vi "InitializeMission.vi"(0 "GenericMission in":refnum<class "GenericMission.lvclass">, 1 "Duration (s)":dbl=-1.0, 5 "Mission Type":T2, 7 "ID#":u16, 9 "Points of Interest":T1[](array[typedef]) {"North" format="%#_10f"; "East" format="%#_8f"}, 11 "Error In":errorcluster, 12 "Timeout (s)":dbl=-1.0, 14 "Tolerance (m)":dbl) -> (4 "GenericMission out":refnum<class "GenericMission.lvclass">, 15 "Error Out":errorcluster)   [LabVIEW 2013, in "GenericMission.lvclass"]
doc: "This VI initializes a mission. Mission Type, Points of Interest, and Tolerance are required, and timeout and duration are both optional. This should not need to be overriden by child classes."
uses:
  GenericMission.lvclass
  Data/TypeDefs/MissionTypeControl.ctl
  Data/TypeDefs/UTM Location.ctl
  GenericMission.lvclass/GenericMission.ctl
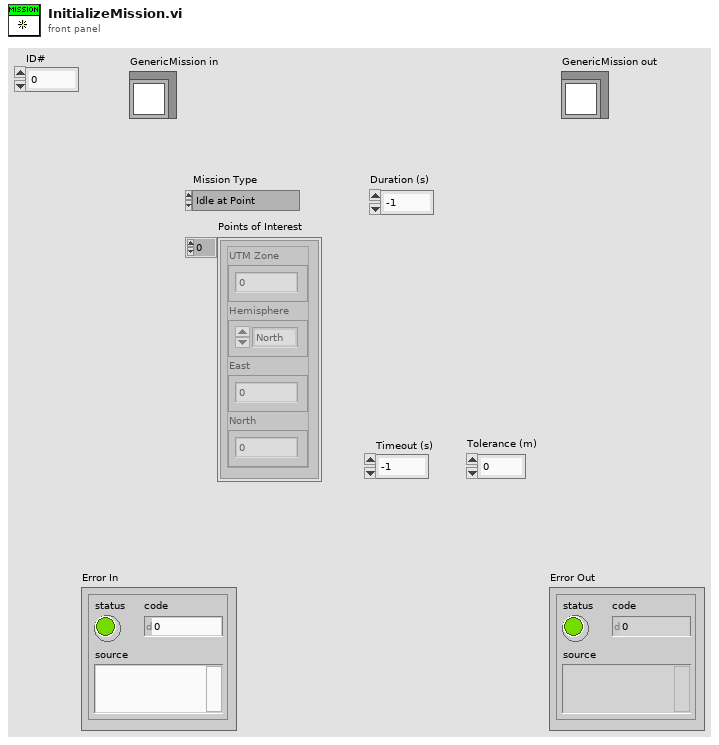
[diagram p1: front panel]
types:
  T1 = typedef "UTM Location.ctl" = cluster{"UTM Zone":dbl, "Hemisphere":enum16{"North", "South"}, "East":dbl, "North":dbl}
  T2 = typedef "MissionTypeControl.ctl" = enum16{"Idle at Point", "Drive to Waypoint", "Round Buoy to Port", "Round Buoy to Starboard", "Pass Between Buoys", "Station Keeping"}
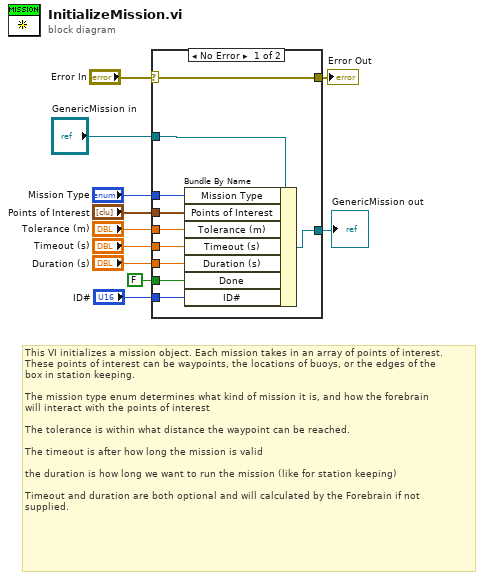
[diagram p0: block diagram]
diagram:
  # "This VI initializes a mission object. Each mission takes in an array of points of interest.\nThese points of interest can be waypoints, the locations of buoys, or the edges of the \nbox in station keeping. \n\nThe mission type enum determines what kind of mission it is, and how the forebrain \nwill interact with the points of interest\n\nThe tolerance is within what distance the waypoint can be reached. \n\nThe timeout is after how long the mission is valid\n\nthe duration is how long we want to run the mission (like for station keeping)\n\nTimeout and duration are both optional and will calculated by the Forebrain if not \nsupplied."
  n1 = case shown="No Error" "Error In" {
    selector: "Error In" -> [w21 w22]
    tunnel: [w21 w22] -> w10
    tunnel: "Mission Type" -> [w20 _]
    tunnel: "Points of Interest" -> [w19 _]
    tunnel: "Tolerance (m)" -> [w18 _]
    tunnel: "Timeout (s)" -> [w17 _]
    tunnel: "Duration (s)" -> [w16 _]
    tunnel: "GenericMission in" -> [w15 w23]
    tunnel: [w14 w23] -> w3
    tunnel: FALSE ("Done") -> [w13 _]
    tunnel: "ID#" -> [w12 _]
    frame No Error {
      n2 = Bundle By Name(cluster=w15, "Mission Type"=w20, "Points of Interest"=w19, "Tolerance (m)"=w18, "Timeout (s)"=w17, "Duration (s)"=w16, "Done"=w13, "ID#"=w12) -> (w14:refnum<class "GenericMission.lvclass">)
    }
    frame Error {
    }
  }
  "Error Out" <- w10
  "GenericMission out" <- w3
